vi "Draw True-Color Pixmap.vi"(0 "picture":picture, 2 "top left point(0, 0)":cluster{"x":i16, "y":i16}, 3 "data (RGB format)":u32[][](array[numeric]) format="%x", 4 "mask":u8[](array[numeric])) -> (6 "new picture":picture)   [LabVIEW 2020]
doc: "Converts a pixmap into a picture so you can use other Picture Functions VIs to append drawing instructions to the image. The data type you wire to the <B>data</B> input determines the polymorphic instance to use. If you want to convert a 4-bit or 8-bit pixmap, you must manually select the polymorphic instance you want to use."
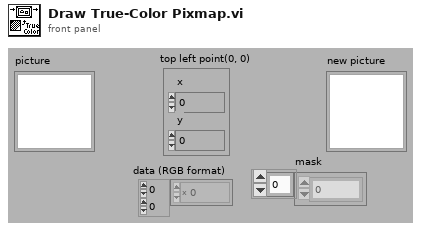
[diagram p1: front panel]
types:
  T1 = typedef "imagedata.ctl" = cluster{"image type":i32, "image depth":i32, "image":u8[], "mask":u8[], "colors":u32[], "Rectangle":cluster{"left":i16, "top":i16, "right":i16, "bottom":i16}}
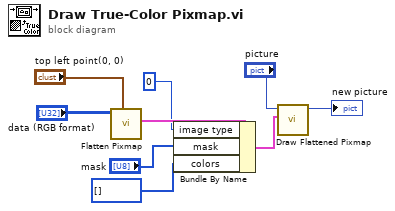
[diagram p0: block diagram]
diagram:
  n1 = call "Flatten Pixmap.vi"("top left"="top left point(0, 0)", "24-bit pixmap"="data (RGB format)") -> ("image data"=w5:T1)  [unwired: 9 in]
  n2 = Bundle By Name(cluster=w5, "image type"=u16 0, "mask"="mask", "colors"=u32[] []) -> (w1:T1)
  n3 = call "Draw Flattened Pixmap.vi"("image data"=w1, "picture"="picture") -> ("new picture"=→"new picture":picture)  [unwired: 7 in]
